vi "FdxCmdEDESubClkControlCvi.vi"(8 "error in":errorcluster, 9 "EDESubClkCntlIn":T1, 10 "EDEScriberHandle":u32, 11 "InstrumentHandle":u32) -> (0 "error out":errorcluster, 2 "EDESubscriberHandleOut":u32, 3 "InstrumentHandle":u32)   [LabVIEW 2020, in "AIM664LV.lvlib"]
doc: "This function is used to control the EDE subscriber Clock."
uses:
  AIM664LV.lvlib
  AFDX_LibraryAdmin/FdxGlobalDllPath.vi
panel:
  out "ClkLow":u32
  out "ClkHigh":u32
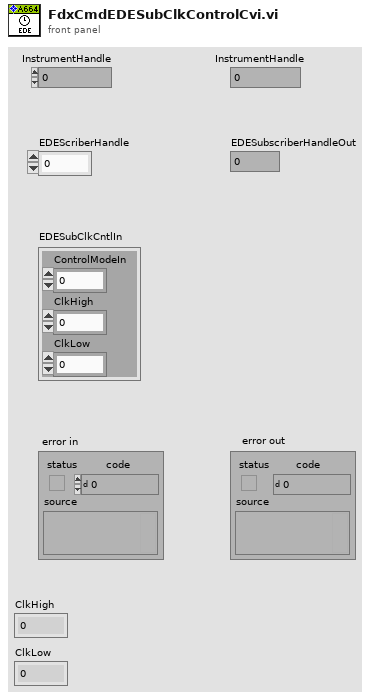
[diagram p1: front panel]
types:
  T1 = cluster{"ControlModeIn":u32, "ClkHigh":u32, "ClkLow":u32}
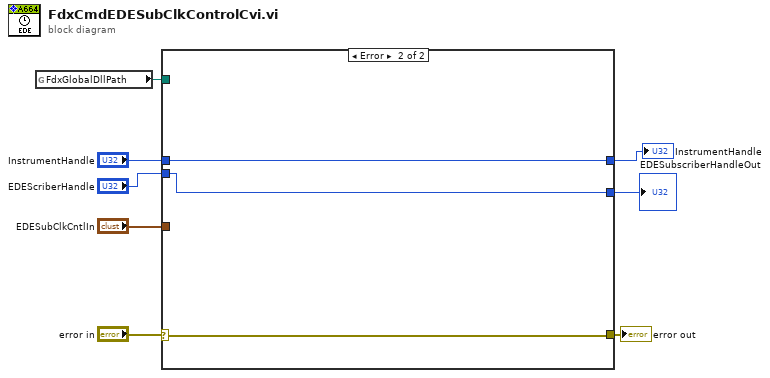
[diagram p0: block diagram]
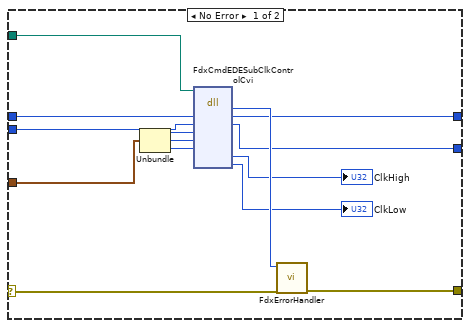
[diagram p2: hidden frame]
diagram:
  n1 = global read "FdxGlobalDllPath.vi" "FdxGlobalDllPath"() -> (w6:path)
  n2 = case shown="Error" "error in" {
    selector: "error in" -> [w21 w25]
    tunnel: [w22 w25] -> w8
    tunnel: w6 -> [w14 _]
    tunnel: "InstrumentHandle" -> [w13 w24]
    tunnel: [w12 w24] -> w4
    tunnel: "EDEScriberHandle" -> [w11 w23]
    tunnel: "EDESubClkCntlIn" -> [w10 _]
    tunnel: [w9 w23] -> w1
    frame No Error {
      n3 = Unbundle(w10) -> ("ControlModeIn"=w17:u32, "ClkHigh"=w16:u32, "ClkLow"=w15:u32)
      n4 = dll-call lib="aim_fdx.19.dll" fn="FdxCmdEDESubClkControlCvi"(path in=w14, "InstrumentHandle"=w13, "EDESubscriberHandle"=w11, "ControlMode"=w17, "ClkHigh"=w16, "ClkLow"=w15) -> ("status"=w20:i32, "InstrumentHandle"=w12:u32, "EDESubscriberHandle"=w9:u32, "ClkHigh"=→"ClkHigh":u32, "ClkLow"=→"ClkLow":u32)  [unwired: 5 in, 4 out]
      n5 = call "FdxErrorHandler.vi"("error in"=w21, "AIM Error"=w20) -> ("error out"=w22:errorcluster)  [unwired: 9 in]
    }
    frame Error {
    }
  }
  "error out" <- w8
  "InstrumentHandle" <- w4
  "EDESubscriberHandleOut" <- w1
